vi "GV_Zoom_Fitsize_PerUnit.vi"(5 "Boolean-id":bool[](array[boolean]), 6 "TypeIdxPerAnalogTag":i32[](array[numeric]), 7 "AutoScale":T1, 8 "IndexPerType":cluster{"EngUnit":string, "IdxPerType":i32[]}[](array[cluster]), 9 "Graph-ref":refnum<vi>, 10 "EngUnitTypes":string[](array[string]), 11 "BooleanPixels":u16) -> (1 "Bottoms":dbl[](array[numeric]), 2 "ScaleIndexes":i32[](array[numeric]), 3 "Tops":dbl[](array[numeric]))   [LabVIEW 2020]
doc: "Determine the stack sizes for a combination of numerical and boolean tags,\nwhen some kind of stacked autoscale is used."
uses:
  controls/AutoScale.ctl
  Gviewer.lvclass
panel:
  out "Error OUT":errorcluster
  in  "error in (no error)":errorcluster
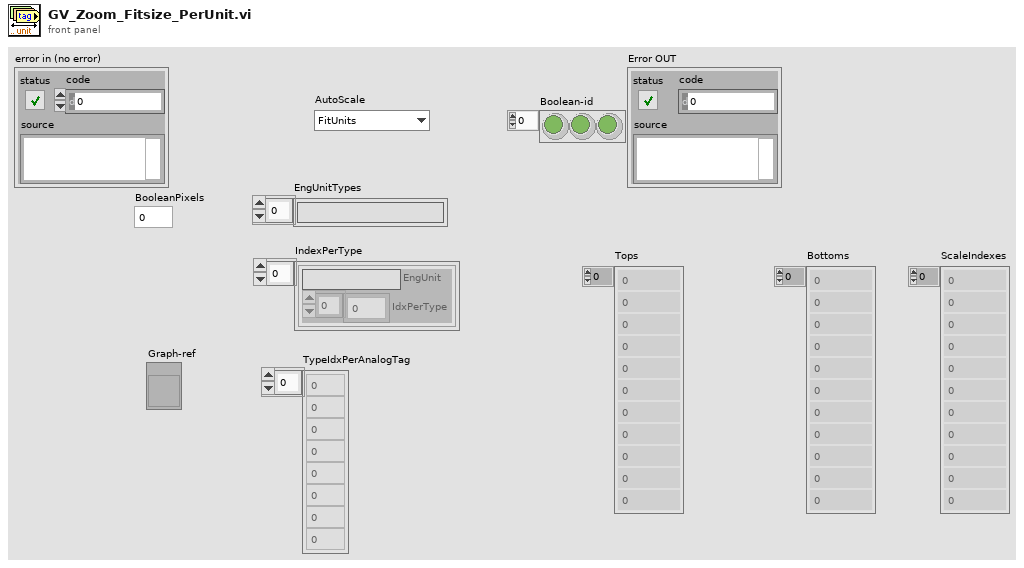
[diagram p1: front panel]
types:
  T1 = typedef "Sgraph_lib_V1.lvlib/Gviewer.lvclass/AutoScale.ctl" = enum16{"FitUnits", "FitAnalogs", "FitAll", "Stack"}
  T2 = typedef "LVRectTypeDef.ctl" = cluster{"Left":i16, "Top":i16, "Right":i16, "Bottom":i16}
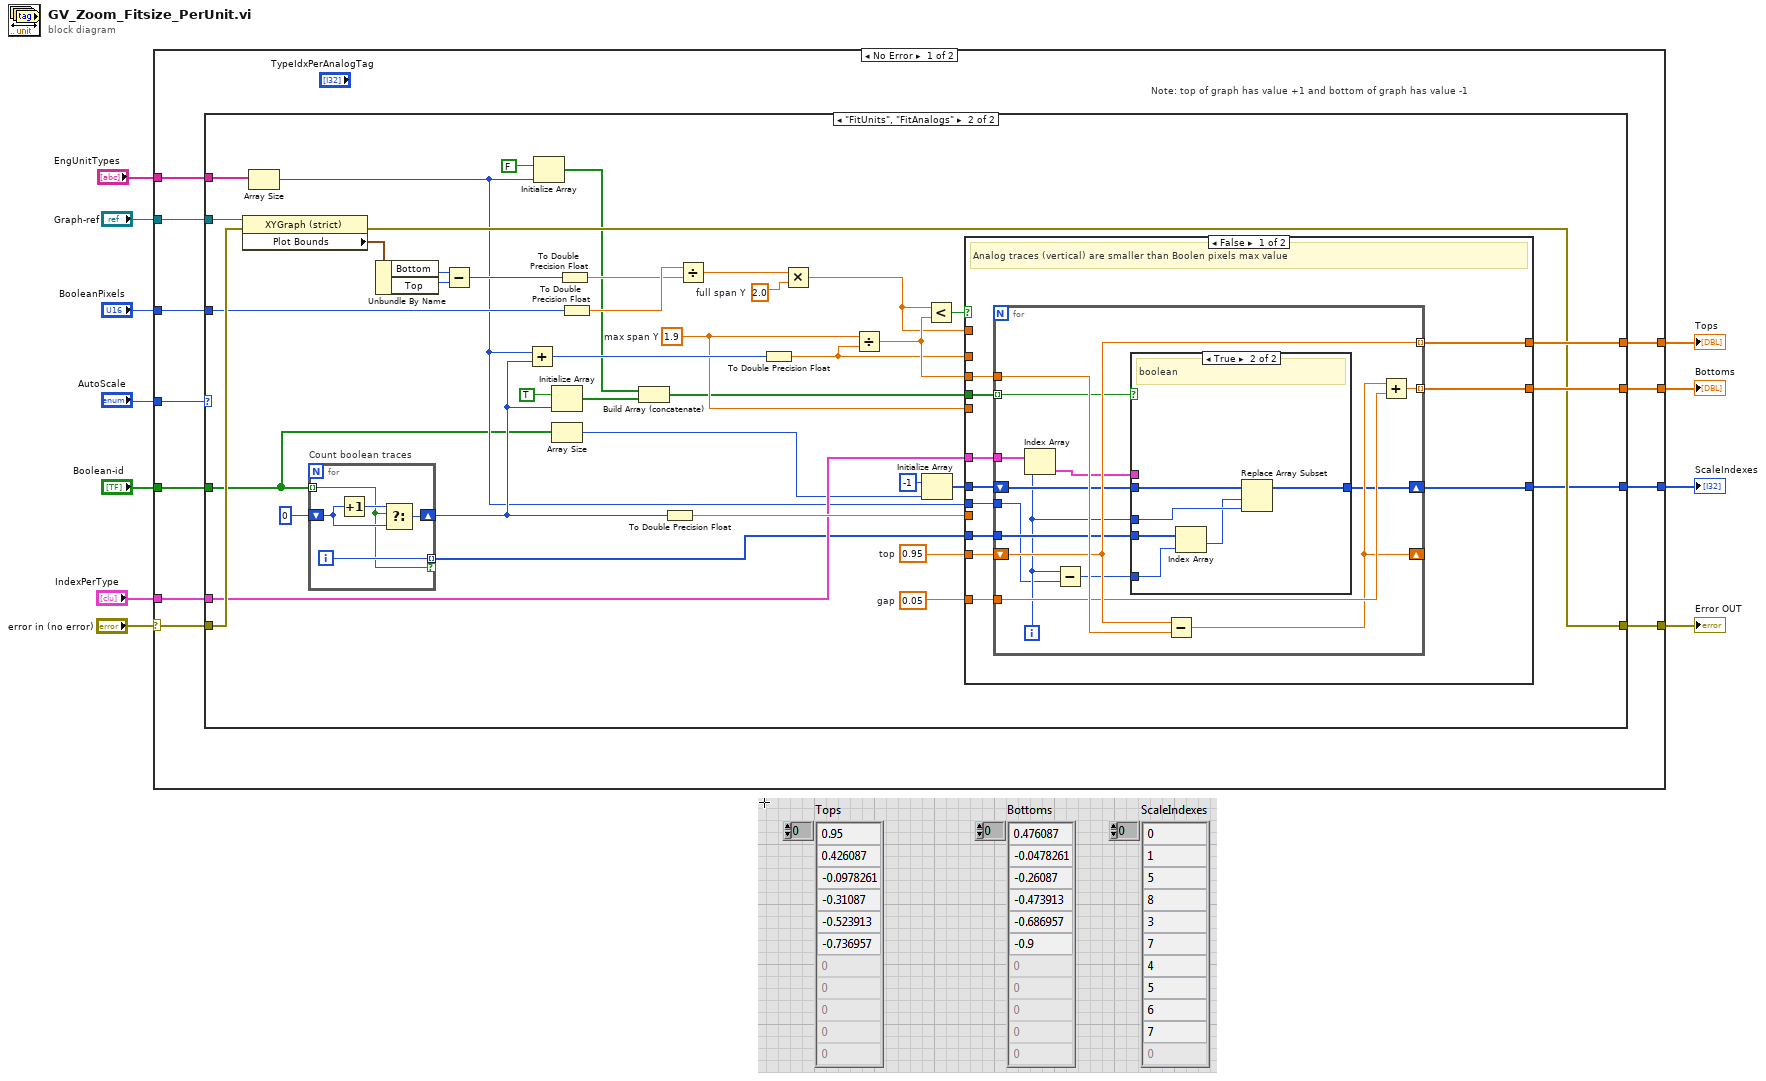
[diagram p0: block diagram]
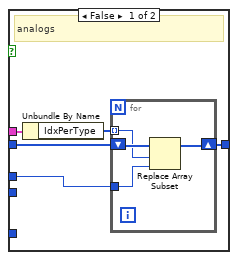
[diagram p3: hidden frame]
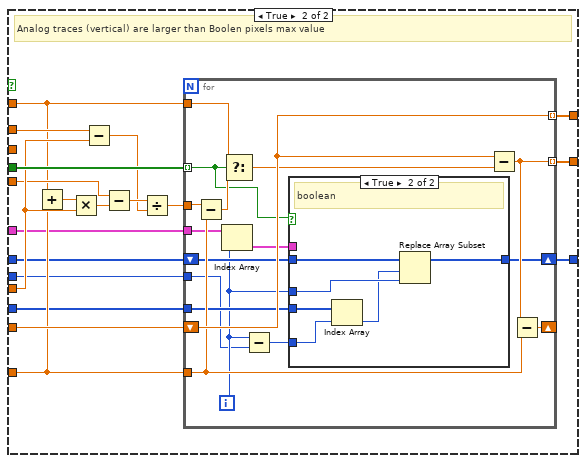
[diagram p4: hidden frame]
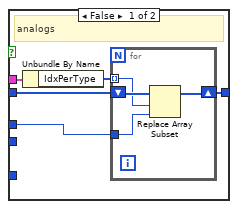
[diagram p5: hidden frame]
diagram:
  n1 = case shown="No Error" "error in (no error)" {
    selector: "error in (no error)" -> [w18 w159]
    tunnel: "Boolean-id" -> [w22 _]
    tunnel: "AutoScale" -> [w21 _]
    tunnel: "BooleanPixels" -> [w20 _]
    tunnel: "Graph-ref" -> [w19 _]
    tunnel: [w17 w159] -> w6
    tunnel: [w16 _] -> w5
    tunnel: [w15 _] -> w4
    tunnel: "EngUnitTypes" -> [w14 _]
    tunnel: [w13 _] -> w2
    tunnel: "IndexPerType" -> [w12 _]
    frame No Error {
      # "Note: top of graph has value +1 and bottom of graph has value -1"
      n2 = case shown="\"FitUnits\", \"FitAnalogs\"" w21 {
        tunnel: w22 -> [_ w27]
        tunnel: w20 -> [_ w48]
        tunnel: w19 -> [_ w59]
        tunnel: w18 -> [w23 w58]
        tunnel: [w23 w51] -> w17
        tunnel: [_ w61] -> w16
        tunnel: [_ w60] -> w15
        tunnel: w14 -> [_ w43]
        tunnel: [_ w31] -> w13
        tunnel: w12 -> [_ w30]
        frame Default {
        }
        frame "FitUnits", "FitAnalogs" {
          w38 = 2.0  # full span Y
          w39 = 1.9  # max span Y
          w56 = 0.05  # gap
          w57 = 0.95  # top
          n3 = property class="XYGraph (strict)"(reference=w59, error in=w58) -> (error out=w51:errorcluster, "Plot Bounds"=w54:T2)  [unwired: 1 out]
          n4 = Array Size(array=w43) -> (size(s)=w29:i32)
          n5 = for "Count boolean traces" {
            tunnel: w27 -> [w154] mode=indexing
            shift-right: [w156] -> w36
            shift-left: 0 ("y") -> [w158]
            tunnel: [w155] -> w24 mode=indexing if=w154
            i -> [w155]
            n6 = Increment(x=w158) -> (x+1=w157:i32)
            n7 = Select(t=w157, s=w154, f=w158) -> (s? t:f=w156:i32)
          }
          n8 = Unbundle By Name(w54) -> ("Bottom"=w53:i16, "Top"=w52:i16)
          n9 = Subtract(x=w53, y=w52) -> (x-y=w49:i16)
          n10 = Add(x=w29, y=w36) -> (x+y=w41:i32)
          n11 = Initialize Array(FALSE, w29) -> (w33:bool[])
          n12 = Initialize Array(TRUE, w36) -> (w34:bool[])
          n13 = Array Size(array=w27) -> (size(s)=w26:i32)
          n14 = To Double Precision Float(number=w49) -> (double precision float=w46:dbl)
          n15 = To Double Precision Float(number=w48) -> (double precision float=w47:dbl)
          n16 = Build Array (concatenate)(w33, w34) -> (w32:bool[])
          n17 = To Double Precision Float(number=w36) -> (double precision float=w42:dbl)
          n18 = Divide(x=w47, y=w46) -> (x/y=w45:dbl)
          n19 = To Double Precision Float(number=w41) -> (double precision float=w40:dbl)
          n20 = Multiply(x=w45, y=w38) -> (x*y=w44:dbl)
          n21 = Divide(x=w39, y=w40) -> (x/y=w50:dbl)
          n22 = Initialize Array(-1 ("Tops"), w26) -> (w25:i32[])
          n23 = Less?(x=w44, y=w50) -> (x < y?=w55:bool)
          n24 = case shown="False" w55 {
            tunnel: w56 -> [w73 w109]
            tunnel: [w72 w121] -> w61
            tunnel: [w71 w120] -> w60
            tunnel: w57 -> [w70 w118]
            tunnel: w40 -> [_ w115]
            tunnel: w44 -> [_ w110]
            tunnel: w50 -> [w69 _]
            tunnel: w32 -> [w68 w119]
            tunnel: w42 -> [_ w112]
            tunnel: w39 -> [_ w111]
            tunnel: w25 -> [w67 w107]
            tunnel: [w66 w106] -> w31
            tunnel: w30 -> [w65 w105]
            tunnel: w29 -> [w64 w104]
            tunnel: w24 -> [w63 w103]
            frame False {
              # "Analog traces (vertical) are smaller than Boolen pixels max value"
              n25 = for {
                tunnel: w73 -> [w85]
                tunnel: [w86] -> w72 mode=indexing
                tunnel: [w83] -> w71 mode=indexing
                shift-right: [w84] -> _
                shift-left: w70 -> [w86]
                tunnel: w69 -> [w87]
                tunnel: w68 -> [w78] mode=indexing
                shift-right: [w80] -> w66
                shift-left: w67 -> [w79]
                tunnel: w65 -> [w82]
                tunnel: w64 -> [w74]
                tunnel: w63 -> [w77]
                i -> [w75]
                n26 = Index Array(array=w82, index=w75) -> (element=w81:cluster{"EngUnit":string, "IdxPerType":i32[]})
                n27 = Subtract(x=w75, y=w74) -> (x-y=w76:i32)
                n28 = case shown="True" w78 {
                  tunnel: w81 -> [w92 _]
                  tunnel: [w90 w101] -> w80
                  tunnel: w79 -> [w91 w102]
                  tunnel: w75 -> [w88 w100]
                  tunnel: w77 -> [_ w99]
                  tunnel: w76 -> [_ w98]
                  frame False {
                    # "analogs"
                    n29 = Unbundle By Name(w92) -> ("IdxPerType"=w89:i32[])
                    n30 = for {
                      shift-right: [w95] -> w90
                      shift-left: w91 -> [w96]
                      tunnel: w89 -> [w94] mode=indexing
                      tunnel: w88 -> [w93]
                      n31 = Replace Array Subset(array=w96, new element=w93, index=w94) -> (w95:i32[])
                    }
                  }
                  frame True {
                    # "boolean"
                    n32 = Index Array(array=w99, index=w98) -> (element=w97:i32)
                    n33 = Replace Array Subset(array=w102, new element=w100, index=w97) -> (w101:i32[])
                  }
                }
                n34 = Subtract(x=w86, y=w87) -> (x-y=w84:dbl)
                n35 = Add(x=w84, y=w85) -> (x+y=w83:dbl)
              }
            }
            frame True {
              # "Analog traces (vertical) are larger than Boolen pixels max value"
              n36 = Add(x=w110, y=w109) -> (x+y=w108:dbl)
              n37 = Multiply(x=w108, y=w112) -> (x*y=w117:dbl)
              n38 = Subtract(x=w115, y=w112) -> (x-y=w114:dbl)
              n39 = Subtract(x=w111, y=w117) -> (x-y=w116:dbl)
              n40 = Divide(x=w116, y=w114) -> (x/y=w113:dbl)
              n41 = for {
                tunnel: w109 -> [w132]
                tunnel: [w138] -> w121 mode=indexing
                tunnel: [w135] -> w120 mode=indexing
                shift-right: [w134] -> _
                shift-left: w118 -> [w138]
                tunnel: w119 -> [w129] mode=indexing
                tunnel: w113 -> [w133]
                tunnel: w110 -> [w136]
                shift-right: [w126] -> w106
                shift-left: w107 -> [w127]
                tunnel: w105 -> [w130]
                tunnel: w104 -> [w123]
                tunnel: w103 -> [w125]
                i -> [w124]
                n42 = Subtract(x=w133, y=w132) -> (x-y=w131:dbl)
                n43 = Index Array(array=w130, index=w124) -> (element=w128:cluster{"EngUnit":string, "IdxPerType":i32[]})
                n44 = Select(t=w136, s=w129, f=w131) -> (s? t:f=w137:dbl)
                n45 = Subtract(x=w124, y=w123) -> (x-y=w122:i32)
                n46 = case shown="True" w129 {
                  tunnel: w128 -> [w143 _]
                  tunnel: [w141 w152] -> w126
                  tunnel: w127 -> [w142 w153]
                  tunnel: w124 -> [w139 w151]
                  tunnel: w125 -> [_ w150]
                  tunnel: w122 -> [_ w149]
                  frame False {
                    # "analogs"
                    n47 = Unbundle By Name(w143) -> ("IdxPerType"=w140:i32[])
                    n48 = for {
                      shift-right: [w146] -> w141
                      shift-left: w142 -> [w147]
                      tunnel: w140 -> [w145] mode=indexing
                      tunnel: w139 -> [w144]
                      n49 = Replace Array Subset(array=w147, new element=w144, index=w145) -> (w146:i32[])
                    }
                  }
                  frame True {
                    # "boolean"
                    n50 = Index Array(array=w150, index=w149) -> (element=w148:i32)
                    n51 = Replace Array Subset(array=w153, new element=w151, index=w148) -> (w152:i32[])
                  }
                }
                n52 = Subtract(x=w138, y=w137) -> (x-y=w135:dbl)
                n53 = Subtract(x=w135, y=w132) -> (x-y=w134:dbl)
              }
            }
          }
        }
      }
    }
    frame Error {
    }
  }
  "Tops" <- w5
  "Bottoms" <- w4
  "Error OUT" <- w6
  "ScaleIndexes" <- w2
